vi "Adjust Magnetic Field.vi"() -> ()   [LabVIEW 2020]
uses:
  Labview Library/Libraries/UT_Utilities/Utilities.lvlib
  Labview Library/Libraries/UT_Utilities/Support/Peak Parameter.ctl
  Labview Library/Libraries/Basic Experiment/Basic Experiment.lvlib
  Labview Library/Libraries/UT_Utilities/Support/Lorentizan Fit Parameter.ctl
  Labview Library/Libraries/Basic Experiment/Pulse CW settings.ctl
panel:
  in  "PS":string
  in  "Theory Right Peak":dbl=1374.5
  in  "Calculate Right Peak":bool
  in  "Theory Left Peak":dbl=1374.5
  in  "Calculate Left Peak":bool
  in  "Add History":bool=TRUE
  in  "History":T2(array[cluster])
  in  "Zero Field Frequency":dbl=1374.5
  in  "Left Peak Settings":T3={"Num Pts"=30, "Start freq"=1350.0, "Stop freq"=1250.0, " dBm"=-12.0, "AutoTrace Before Exp"=FALSE, "RepoSave"=FALSE, "Pulse Time"=5.8e-08, "Peak Num Limit "=10, "Loop per Update"=10000, "RatioThre"=0.04, "UpdateTime"=20000} {"UpdateTime" format="%.0p"; "Loop per Update" format="%#_6p"; "Pulse Time" format="%#_6p"}
  out "CW Left":cluster{"x":dbl[], "y":dbl[]}[](graph)
  in  "Left Fit Parameter":T4={"Background"=nan, "Peaks Parameter"=[]}
  in  "Right Fit Parameter":T4={"Background"=nan, "Peaks Parameter"=[]}
  out "CW Right":cluster{"x":dbl[], "y":dbl[]}[](graph)=[{"x"=[1550.0, 1553.3333333333333, 1556.6666666666667, 1560.0, 1563.3333333333333, 1566.6666666666667, 1570.0, 1573.3333333333333, 1576.6666666666667, 1580.0, 1583.3333333333333, 1586.6666666666667, 1590.0, 1593.3333333333333, 1596.6666666666667, 1600.0, 1603.3333333333333, 1606.6666666666667, 1610.0, 1613.3333333333333, 1616.6666666666667, 1620.0, 1623.3333333333333, 1626.6666666666667, 1630.0, 1633.3333333333333, 1636.6666666666667, 1640.0, 1643.3333333333333, 1646.6666666666667, 1650.0], "y"=[-0.0013790156547410946, 0.005439216752787599, 0.0030515063168124394, 0.00852491366551554, 0.0034384633625800334, -0.004931043966838238, -0.00019702492365284208, 0.00985823852993947, -0.010230824484090777, -0.0029703163777773435, -0.011223630344935655, -0.005334387039415193, -0.008794466403162055, -0.008557913125404833, -0.00019875183845450572, -0.0037974185424209037, -0.011997800730471665, 0.0038996880249580032, -0.007767679356504939, -0.00567900745988088, 0.0017381228273464658, -0.0050780703332733565, 0.007780689377141705, -0.002619289340101523, 0.005669049017027394, 0.006739629018629542, -0.004387801910688286, -0.008365326328551222, -0.0010899622550107986, 0.009556341751047132, 0.01102533610142503]}, {"x"=array[301 elements], "y"=[nan, nan, nan, nan, nan, nan, nan, nan, nan, nan, nan, nan, nan, nan, nan, nan, nan, nan, nan, nan, nan, nan, nan, nan, nan, nan, nan, nan, nan, nan, nan, nan, nan, nan, nan, nan, nan, nan, nan, nan, nan, nan, nan, nan, nan, nan, nan, nan, nan, nan, nan, nan, nan, nan, nan, nan, nan, nan, nan, nan, nan, nan, nan, nan, nan, nan, nan, nan, nan, nan, nan, nan, nan, nan, nan, nan, nan, nan, nan, nan, nan, nan, nan, nan, nan, nan, nan, nan, nan, nan, nan, nan, nan, nan, nan, nan, nan, nan, nan, nan, nan, nan, nan, nan, nan, nan, nan, nan, nan, nan, nan, nan, nan, nan, nan, nan, nan, nan, nan, nan, nan, nan, nan, nan, nan, nan, nan, nan, nan, nan, nan, nan, nan, nan, nan, nan, nan, nan, nan, nan, nan, nan, nan, nan, nan, nan, nan, nan, nan, nan, nan, nan, nan, nan, nan, nan, nan, nan, nan, nan, nan, nan, nan, nan, nan, nan, nan, nan, nan, nan, nan, nan, nan, nan, nan, nan, nan, nan, nan, nan, nan, nan, nan, nan, nan, nan, nan, nan, nan, nan, nan, nan, nan, nan, nan, nan, nan, nan, nan, nan, nan, nan, nan, nan, nan, nan, nan, nan, nan, nan, nan, nan, nan, nan, nan, nan, nan, nan, nan, nan, nan, nan, nan, nan, nan, nan, nan, nan, nan, nan, nan, nan, nan, nan, nan, nan, nan, nan, nan, nan, nan, nan, nan, nan, nan, nan, nan, nan, nan, nan, nan, nan, nan, nan, nan, nan, nan, nan, nan, nan, nan, nan, nan, nan, nan, nan, nan, nan, nan, nan, nan, nan, nan, nan, nan, nan, nan, nan, nan, nan, nan, nan, nan, nan, nan, nan, nan, nan, nan, nan, nan, nan, nan, nan, nan, nan, nan, nan, nan, nan, nan]}]
  in  "Right Peak Settings":T3={"Num Pts"=30, "Start freq"=1550.0, "Stop freq"=1650.0, " dBm"=-12.0, "AutoTrace Before Exp"=FALSE, "RepoSave"=FALSE, "Pulse Time"=5.8e-08, "Peak Num Limit "=10, "Loop per Update"=10000, "RatioThre"=0.02, "UpdateTime"=20000} {"UpdateTime" format="%.0p"; "Loop per Update" format="%#_6p"; "Pulse Time" format="%#_6p"}
  in  "Left Peak":bool=TRUE
  in  "Right Peak":bool
  in  "stop":bool
  in  "Enqueue Element":bool
  # "Pulse CW Settings"
  # "Pulse CW Settings"
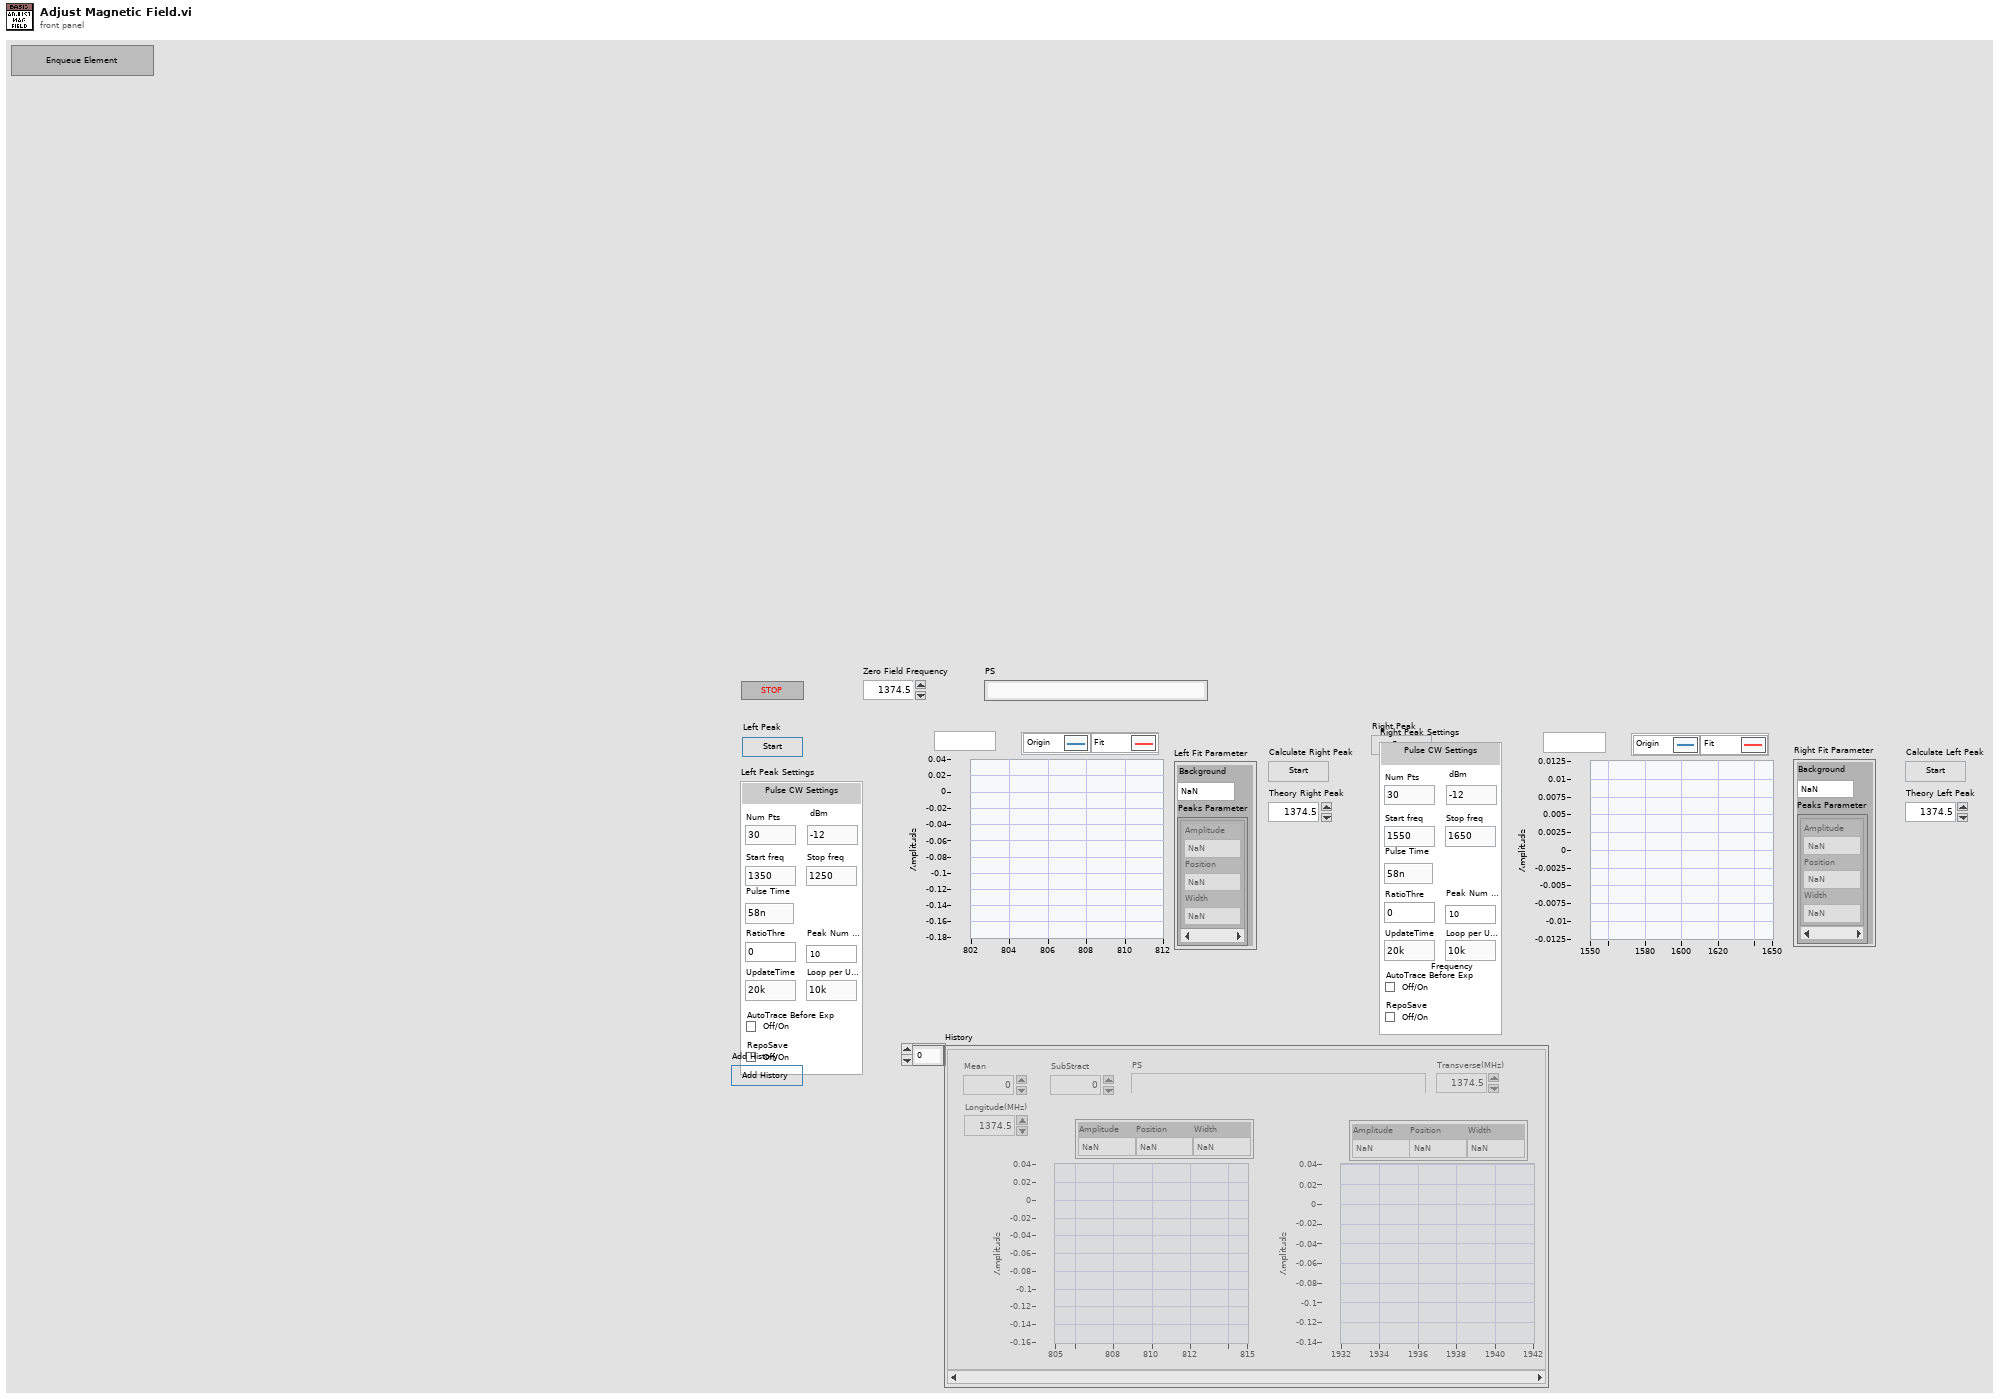
[diagram p1: front panel]
types:
  T1 = typedef "Utilities.lvlib/Peak Parameter.ctl" = cluster{"Amplitude":dbl, "Position":dbl, "Width":dbl}
  T2 = cluster{"Mean":dbl, "SubStract":dbl, "PS":string, "CW Left":cluster{"x":dbl[], "y":dbl[]}[], "CW Right":cluster{"x":dbl[], "y":dbl[]}[], "Left Peak Parameter":T1, "Right Peak Parameter":T1, "Longitude(MHz)":dbl, "Transverse(MHz)":dbl}[]
  T3 = typedef "Basic Experiment.lvlib/Pulse CW settings.ctl" = cluster{"Num Pts":i32, "Start freq":dbl, "Stop freq":dbl, " dBm":dbl, "AutoTrace Before Exp":bool, "RepoSave":bool, "Pulse Time":dbl, "Peak Num Limit ":i32, "Loop per Update":u32, "RatioThre":dbl, "UpdateTime":i32}
  T4 = typedef "Utilities.lvlib/Lorentizan Fit Parameter.ctl" = cluster{"Background":dbl, "Peaks Parameter":T1[]}
  T5 = cluster{"Mean":dbl, "SubStract":dbl, "PS":string, "CW Left":cluster{"x":dbl[], "y":dbl[]}[], "CW Right":cluster{"x":dbl[], "y":dbl[]}[], "Left Peak Parameter":T1, "Right Peak Parameter":T1, "Longitude(MHz)":dbl, "Transverse(MHz)":dbl}
  T6 = typedef "Basic Experiment.lvlib/CW Results.ctl" = cluster{"Fit Frequency":T7, "Pro":dbl[], "Error Bar":dbl[], "Raw Data Path":path, "Image Path":path}
  T7 = typedef "Basic Experiment.lvlib/CW Fit Frequency.ctl" = cluster{"Fre2":cluster{"Amplitude":dbl, "Position":dbl, "Width":dbl}, "Fre1":cluster{"Amplitude":dbl, "Position":dbl, "Width":dbl}, "Fre3":cluster{"Amplitude":dbl, "Position":dbl, "Width":dbl}, "Background":dbl}
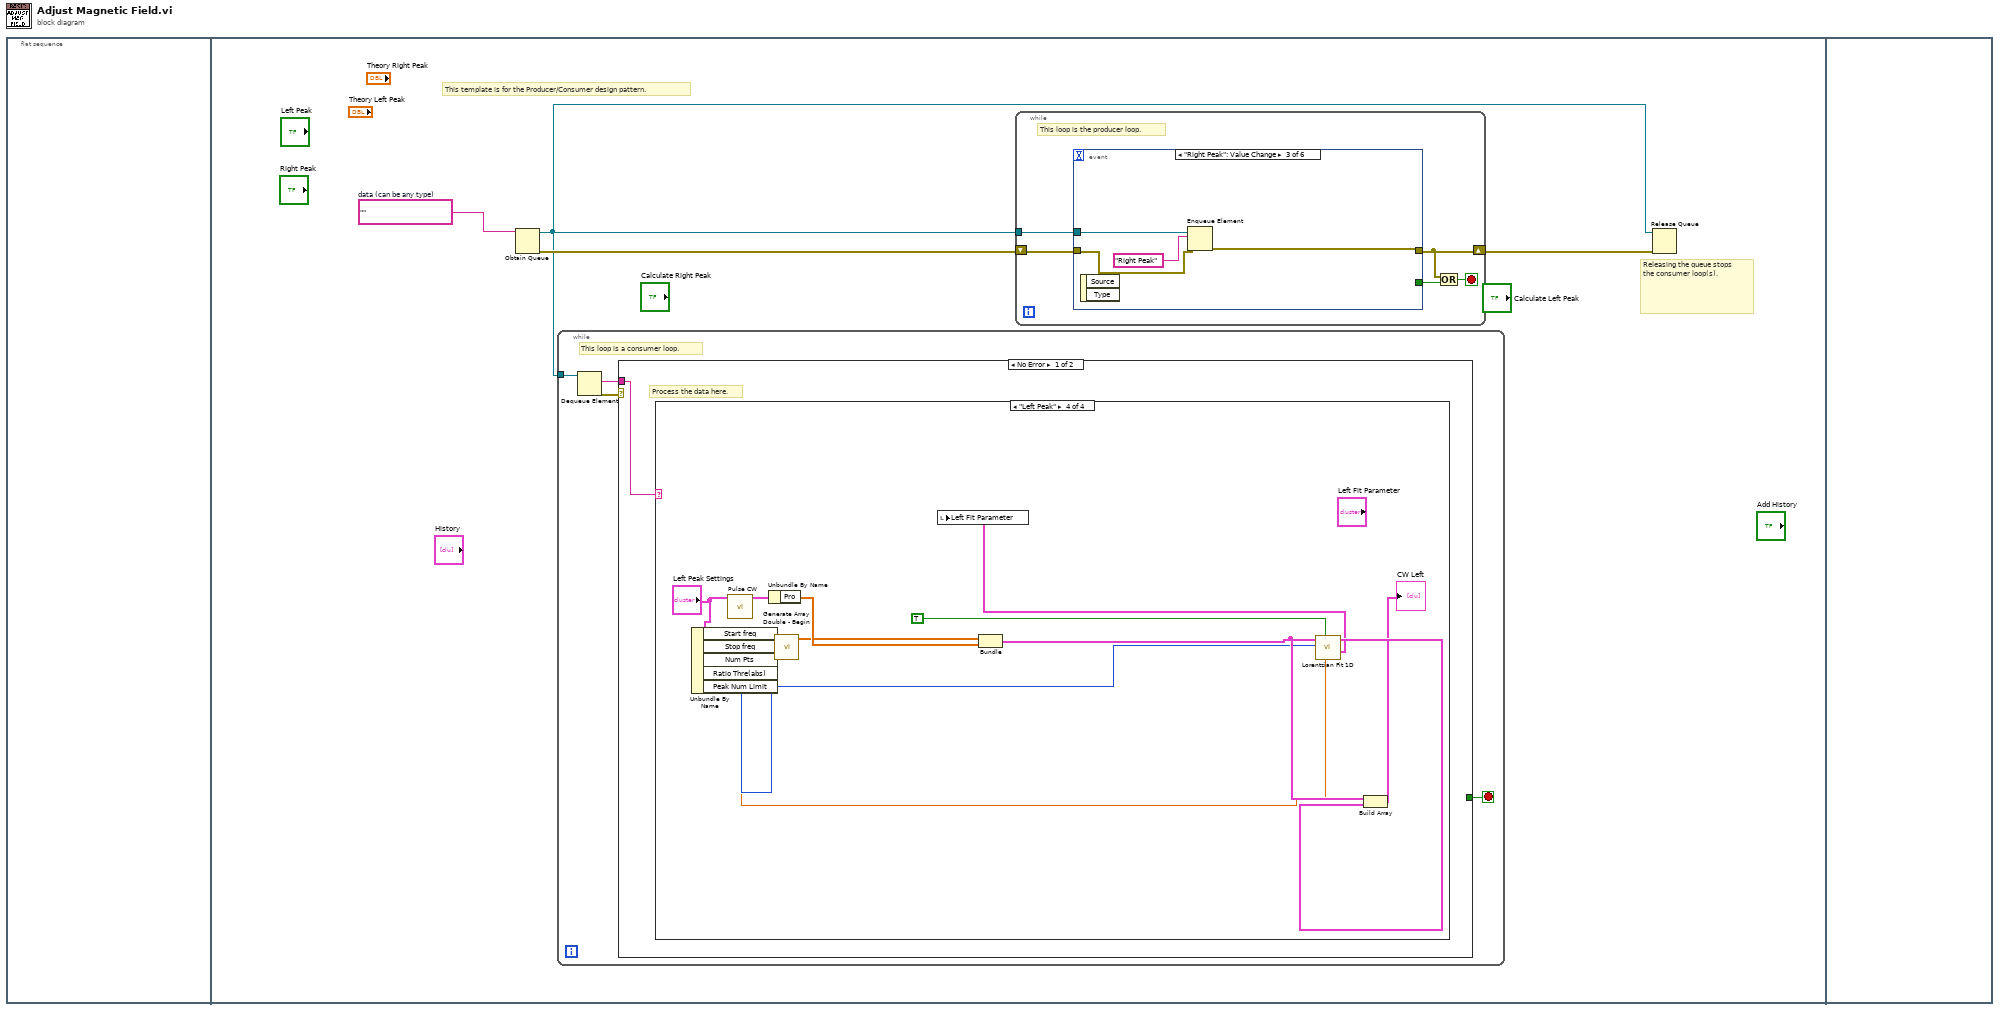
[diagram p0: block diagram]
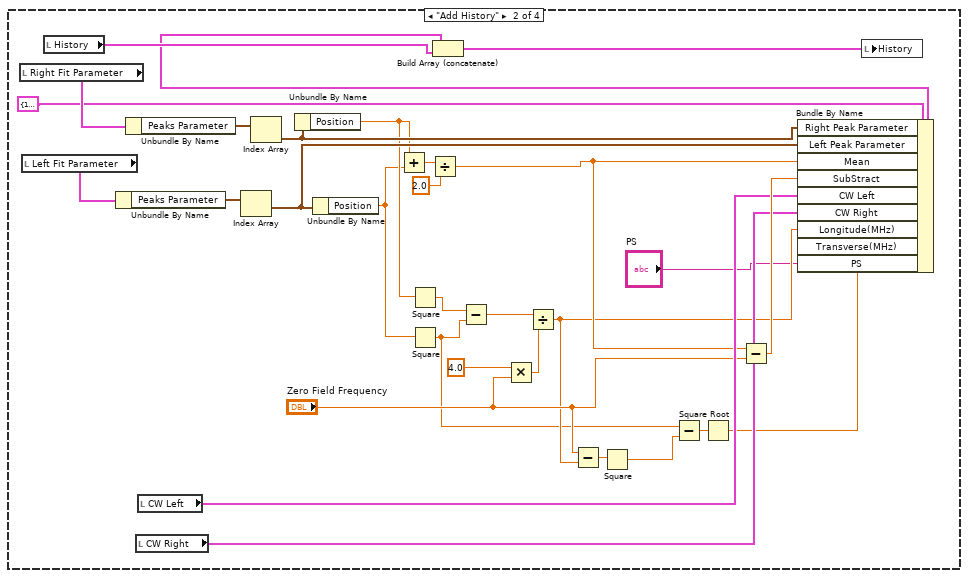
[diagram p3: hidden frame]
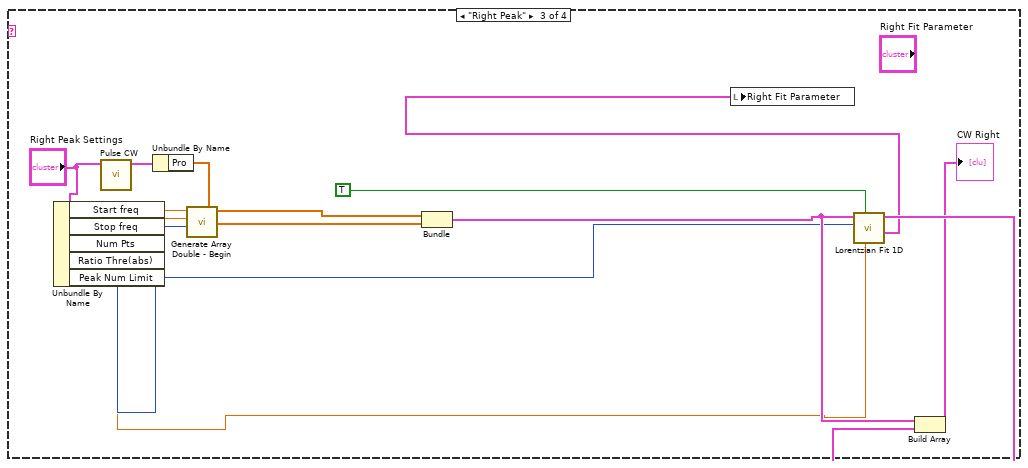
[diagram p4: hidden frame]
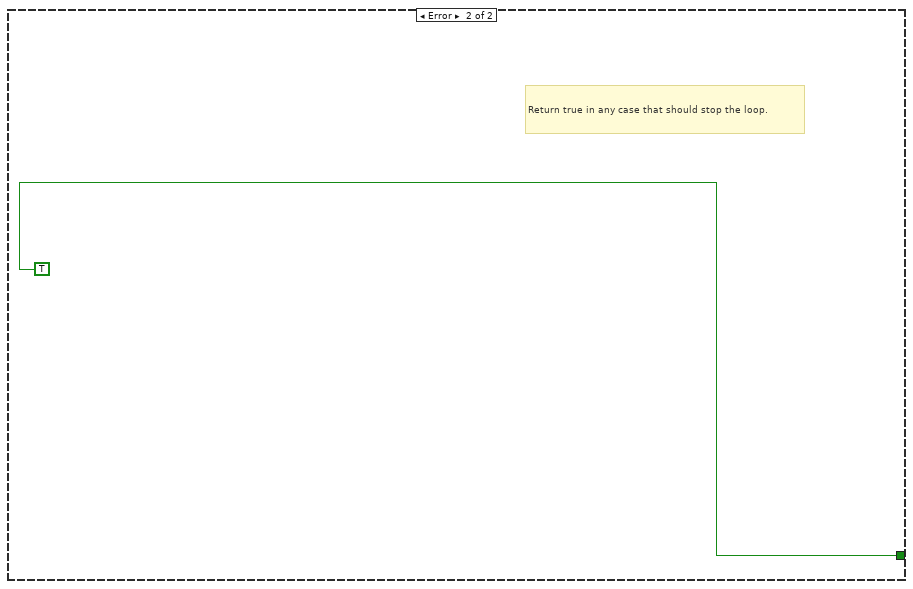
[diagram p5: hidden frame]
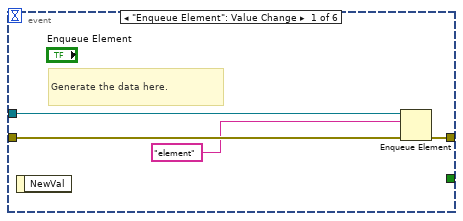
[diagram p6: hidden frame]
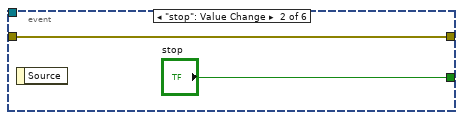
[diagram p7: hidden frame]
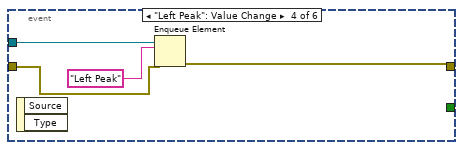
[diagram p8: hidden frame]
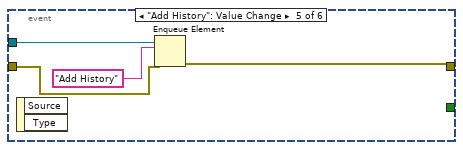
[diagram p9: hidden frame]
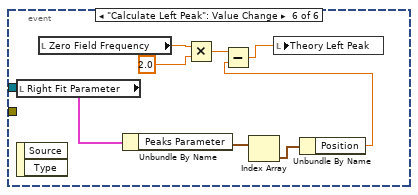
[diagram p10: hidden frame]
diagram:
  n1 = flat-sequence {
    frame #0 {
    }
    frame #1 {
      w2 = ""  # data (can be any type)
      # "Releasing the queue stops the consumer loop(s)."
      # "This template is for the Producer/Consumer design pattern."
      n2 = Obtain Queue(element data type=w2) -> (queue out=w1:refnum<queue>, error out=w4:errorcluster)  [unwired: 4 in, 1 out]
      n3 = while {
        tunnel: w1 -> [w8]
        stop <- w5 stop-if-true
        # "This loop is a consumer loop."
        n4 = Dequeue Element(queue=w8) -> (element=w6:string, error out=w7:errorcluster)  [unwired: 2 in, 2 out]
        n5 = case shown="No Error" w7 {
          tunnel: w6 -> [w9 _]
          tunnel: [_ TRUE] -> w5
          frame No Error {
            # "Process the data here."
            n6 = case shown="\"Left Peak\"" w9 {
              frame "False", Default {
              }
              frame "Add History" {
                n7 = local read "Right Fit Parameter"() -> (w36:T4)
                n8 = local read "Left Fit Parameter"() -> (w39:T4)
                n9 = local read "History"() -> (w31:T2)
                n10 = Unbundle By Name(w39) -> ("Peaks Parameter"=w38:T1[])
                n11 = Unbundle By Name(w36) -> ("Peaks Parameter"=w37:T1[])
                n12 = local read "CW Right"() -> (w28:cluster{"x":dbl[], "y":dbl[]}[])
                n13 = local read "CW Left"() -> (w29:cluster{"x":dbl[], "y":dbl[]}[])
                n14 = Index Array(array=w38) -> (element=w25:T1)  [unwired: 1 in]
                n15 = Index Array(array=w37) -> (element=w24:T1)  [unwired: 1 in]
                n16 = Unbundle By Name(w24) -> ("Position"=w23:dbl)
                n17 = Unbundle By Name(w25) -> ("Position"=w14:dbl)
                n18 = Add(x=w23, y=w14) -> (x+y=w35:dbl)
                n19 = Square(x=w23) -> (x^2=w22:dbl)
                n20 = Square(x=w14) -> (x^2=w11:dbl)
                n21 = Divide(x=w35, y=2.0) -> (x/y=w26:dbl)
                n22 = Subtract(x=w22, y=w11) -> (x-y=w21:dbl)
                n23 = Multiply(x=4.0, y="Zero Field Frequency") -> (x*y=w19:dbl)
                n24 = Divide(x=w21, y=w19) -> (x/y=w17:dbl)
                n25 = Subtract(x="Zero Field Frequency", y=w17) -> (x-y=w16:dbl)
                n26 = Square(x=w16) -> (x^2=w15:dbl)
                n27 = Subtract(x=w11, y=w15) -> (x-y=w13:dbl)
                n28 = Square Root(x=w13) -> (sqrt(x)=w12:dbl)
                n29 = Subtract(x=w26, y="Zero Field Frequency") -> (x-y=w33:dbl)
                n30 = Bundle By Name(cluster=T5 {"Mean"=1414.1094924647537, "SubStract"=39.60949246475366, "PS"="", "CW Left"=[], "CW Right"=[], "Left Peak Parameter"={"Amplitude"=-0.05552543645018247, "Position"=1349.4629709624935, "Width"=6.25}, "Right Peak Parameter"={"Amplitude"=-0.09115089462235382, "Position"=1478.7560139670136, "Width"=6.817754325190208}, "Longitude(MHz)"=nan, "Transverse(MHz)"=nan} ("History"), "Right Peak Parameter"=w24, "Left Peak Parameter"=w25, "Mean"=w26, "SubStract"=w33, "CW Left"=w29, "CW Right"=w28, "Longitude(MHz)"=w17, "Transverse(MHz)"=w12, "PS"="PS") -> (w30:T5)
                n31 = Build Array (concatenate)(w30, w31) -> (w32:T2)
                n32 = local write "History"(w32) -> ()
              }
              frame "Right Peak" {
                n33 = Unbundle By Name("Right Peak Settings") -> ("Start freq"=w49:dbl, "Stop freq"=w48:dbl, "Num Pts"=w47:i32, "Ratio Thre(abs)"=w42:dbl, "Peak Num Limit"=w40:i32)
                n34 = call "Pulse CW.vi"("Settings"="Right Peak Settings") -> ("CW Result"=w51:T6)  [unwired: 8 in, 2 out]
                n35 = Unbundle By Name(w51) -> ("Pro"=w50:dbl[])
                n36 = call "Generate Array Double - Begin.vi"("num of step"=w47, "end"=w48, "begin"=w49) -> ("output array"=w45:dbl[])  [unwired: 5 in, 3 out]
                n37 = Bundle("output array"=w45, "Pro"=w50) -> (w44:cluster{"output array":dbl[], "Pro":dbl[]})  [unwired: 1 in]
                n38 = call "Lorentzian Fit 1D.vi"("Amplitude Limit (0.05)"=w42, "Reverse Peak?"=TRUE, "Peak Number Limit (10)"=w40, "Data"=w44) -> ("Best Fit Parameter"=w41:T4, "Fit Result"=w53:cluster{"x":dbl[], "y":dbl[]})  [unwired: 3 in, 3 out]
                n39 = local write "Right Fit Parameter"(w41) -> ()
                n40 = Build Array(w44, w53) -> (→"CW Right":cluster{"x":dbl[], "y":dbl[]}[])
              }
              frame "Left Peak" {
                n41 = Unbundle By Name("Left Peak Settings") -> ("Start freq"=w63:dbl, "Stop freq"=w62:dbl, "Num Pts"=w61:i32, "Ratio Thre(abs)"=w56:dbl, "Peak Num Limit"=w54:i32)
                n42 = call "Pulse CW.vi"("Settings"="Left Peak Settings") -> ("CW Result"=w65:T6)  [unwired: 8 in, 2 out]
                n43 = Unbundle By Name(w65) -> ("Pro"=w64:dbl[])
                n44 = call "Generate Array Double - Begin.vi"("num of step"=w61, "end"=w62, "begin"=w63) -> ("output array"=w59:dbl[])  [unwired: 5 in, 3 out]
                n45 = Bundle("output array"=w59, "Pro"=w64) -> (w58:cluster{"output array":dbl[], "Pro":dbl[]})  [unwired: 1 in]
                n46 = call "Lorentzian Fit 1D.vi"("Amplitude Limit (0.05)"=w56, "Reverse Peak?"=TRUE, "Peak Number Limit (10)"=w54, "Data"=w58) -> ("Best Fit Parameter"=w55:T4, "Fit Result"=w67:cluster{"x":dbl[], "y":dbl[]})  [unwired: 3 in, 3 out]
                n47 = local write "Left Fit Parameter"(w55) -> ()
                n48 = Build Array(w58, w67) -> (→"CW Left":cluster{"x":dbl[], "y":dbl[]}[])
              }
            }
          }
          frame Error {
            # "Return true in any case that should stop the loop."
          }
        }
      }
      n49 = while {
        shift-right: [w69] -> w3
        shift-left: w4 -> [w72]
        tunnel: w1 -> [w73]
        stop <- w70 stop-if-true
        # "This loop is the producer loop."
        n50 = event shown="[2] \"Right Peak\": Value Change" {
          selector: _ -> [_ _ _ _ _ _]
          dyn-events: _ -> [_ _ _ _ _ _]
          timeout: _ -> [_ _ _ _ _ _]
          tunnel: w73 -> [w77 _ w82 w86 w90 _]
          tunnel: w72 -> [w76 w78 w81 w85 w89 _]
          tunnel: [w75 w78 w80 w84 w88 _] -> w69
          tunnel: [_ "stop" _ _ _ _] -> w71
          event "Enqueue Element": Value Change {
            # "Generate the data here."
            n51 = event-data() -> ()  [unwired: 1 in, 1 out]
            n52 = Enqueue Element(queue=w77, element="element", error in (no error)=w76) -> (error out=w75:errorcluster)  [unwired: 1 in, 2 out]
          }
          event "stop": Value Change {
            n53 = event-data() -> ()  [unwired: 1 in, 1 out]
          }
          event "Right Peak": Value Change {
            n54 = event-data() -> ()  [unwired: 1 in, 2 out]
            n55 = Enqueue Element(queue=w82, element="Right Peak", error in (no error)=w81) -> (error out=w80:errorcluster)  [unwired: 1 in, 2 out]
          }
          event "Left Peak": Value Change {
            n56 = event-data() -> ()  [unwired: 1 in, 2 out]
            n57 = Enqueue Element(queue=w86, element="Left Peak", error in (no error)=w85) -> (error out=w84:errorcluster)  [unwired: 1 in, 2 out]
          }
          event "Add History": Value Change {
            n58 = event-data() -> ()  [unwired: 1 in, 2 out]
            n59 = Enqueue Element(queue=w90, element="Add History", error in (no error)=w89) -> (error out=w88:errorcluster)  [unwired: 1 in, 2 out]
          }
          event "Calculate Left Peak": Value Change {
            n60 = local read "Right Fit Parameter"() -> (w95:T4)
            n61 = event-data() -> ()  [unwired: 1 in, 2 out]
            n62 = local read "Zero Field Frequency"() -> (w99:dbl)
            n63 = Unbundle By Name(w95) -> ("Peaks Parameter"=w96:T1[])
            n64 = Multiply(x=w99, y=2.0) -> (x*y=w97:dbl)
            n65 = Index Array(array=w96) -> (element=w94:T1)  [unwired: 1 in]
            n66 = Unbundle By Name(w94) -> ("Position"=w93:dbl)
            n67 = Subtract(x=w97, y=w93) -> (x-y=w92:dbl)
            n68 = local write "Theory Left Peak"(w92) -> ()
          }
        }
        n69 = Or(x=w69, y=w71) -> (x .or. y?=w70:bool)
      }
      n70 = Release Queue(queue=w1, error in (no error)=w3) -> ()  [unwired: 1 in, 3 out]
    }
    frame #2 {
    }
  }
